vi "Configure TSP Net Connection Characteristics.vi"(8 "error in (no error)":errorcluster, 9 "Wait Time (20 S)":dbl=20.0, 10 "Send Abort Message (T: Enable)":bool=TRUE, 11 "VISA resource name":refnum<visa-resource-name>) -> (0 "error out":errorcluster, 3 "VISA resource name out":refnum<visa-resource-name>)   [LabVIEW 2020, in "Keithley 2600 Series.lvlib"]
doc: "Configures the basic settings for TSP net connection."
uses:
  <instrlib>/Keithley 2600 Series/Keithley 2600 Series.lvlib
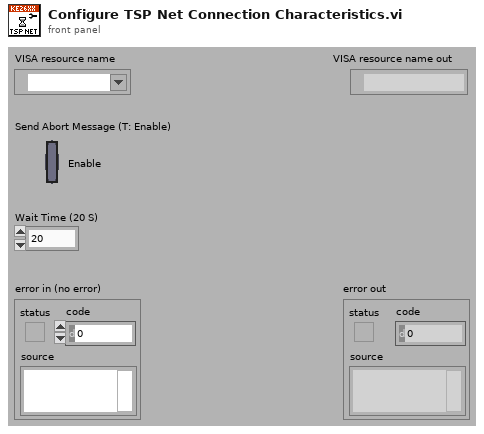
[diagram p1: front panel]
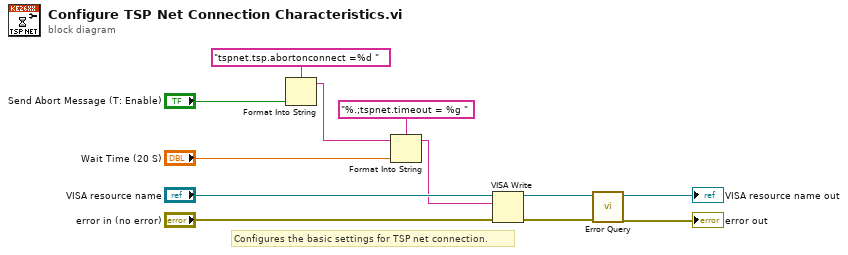
[diagram p0: block diagram]
diagram:
  # "Configures the basic settings for TSP net connection."
  n1 = Format Into String(format string="tspnet.tsp.abortonconnect =%d ", "Send Abort Message (T: Enable)") -> (resulting string=w2:string)  [unwired: 2 in, 1 out]
  n2 = Format Into String(format string="%.;tspnet.timeout = %g ", initial string=w2, "Wait Time (20 S)") -> (resulting string=w1:string)  [unwired: 1 in, 1 out]
  n3 = VISA Write(VISA resource name="VISA resource name", write buffer=w1, error in (no error)="error in (no error)") -> (VISA resource name out=w8:refnum<visa-resource-name>, error out=w7:errorcluster)  [unwired: 1 out]
  n4 = call <instrlib>:"Error Query.vi"("error in (no error)"=w7, "VISA resource name"=w8) -> ("error out"=→"error out":errorcluster, "VISA resource name out"=→"VISA resource name out":refnum<visa-resource-name>)  [unwired: 6 in, 2 out]
